vi "CRYCalc Constant Unit.vi"(6 "B_axis mode":u16(slide) scale=0.0..2.0, 7 "A_axis mode":u16(slide) scale=0.0..2.0, 8 "Work in":u16(slide), 9 "Operator":u16(ring) items=["+", "--", "x", "/"], 10 "B data for units":T1={"Name"="", "Curve"=[], "X data"=1, "Y data"=1, "Z data"=1, "X axis"=0, "Y axis"=1, "Z axis"=1, "X unit"="Hz", "Y unit"="", "Z unit"="deg.", "X dB ref"=1.0, "Y dB ref"=1.0, "Z dB ref"=1.0, "single val"=FALSE, "protected"=FALSE, "display X"=TRUE, "display Y"=TRUE, "display Z"=TRUE, "Test Info"="", "Step No."=0, "Plot Settings"={"Color"=0, "Interpolation"=0, "Point Style"=0, "Line Style"=0, "Point Color"=0, "Line Width"=0, "Bar Plot Style"=0, "Fill To"=0}, "AutoProtect"=FALSE} {"Z data" items=["dB", "Lin"]; "X data" items=["dB", "Lin"]; "Y data" items=["dB", "Lin"]; "Z dB ref" format="%.1f"; "Z axis" items=["Log", "Lin"]; "X dB ref" format="%.1f"; "X axis" items=["Log", "Lin"]; "Y axis" items=["Log", "Lin"]; "Y dB ref" format="%.1f"; "Curve"."z" format="%.2f"; "Curve"."y" format="%.2f"; "Curve"."x" format="%.2f"}, 11 "A data for units":T1={"Name"="", "Curve"=[], "X data"=1, "Y data"=1, "Z data"=1, "X axis"=0, "Y axis"=1, "Z axis"=1, "X unit"="Hz", "Y unit"="", "Z unit"="deg.", "X dB ref"=1.0, "Y dB ref"=1.0, "Z dB ref"=1.0, "single val"=FALSE, "protected"=FALSE, "display X"=TRUE, "display Y"=TRUE, "display Z"=TRUE, "Test Info"="", "Step No."=0, "Plot Settings"={"Color"=0, "Interpolation"=0, "Point Style"=0, "Line Style"=0, "Point Color"=0, "Line Width"=0, "Bar Plot Style"=0, "Fill To"=0}, "AutoProtect"=FALSE} {"Z data" items=["dB", "Lin"]; "X data" items=["dB", "Lin"]; "Y data" items=["dB", "Lin"]; "Z dB ref" format="%.1f"; "Z axis" items=["Log", "Lin"]; "X dB ref" format="%.1f"; "X axis" items=["Log", "Lin"]; "Y axis" items=["Log", "Lin"]; "Y dB ref" format="%.1f"; "Curve"."z" format="%.2f"; "Curve"."y" format="%.2f"; "Curve"."x" format="%.2f"}) -> (3 "Result out":T1={"Name"="", "Curve"=[], "X data"=1, "Y data"=1, "Z data"=1, "X axis"=0, "Y axis"=1, "Z axis"=1, "X unit"="Hz", "Y unit"="", "Z unit"="deg.", "X dB ref"=1.0, "Y dB ref"=1.0, "Z dB ref"=1.0, "single val"=FALSE, "protected"=FALSE, "display X"=TRUE, "display Y"=TRUE, "display Z"=TRUE, "Test Info"="", "Step No."=0, "Plot Settings"={"Color"=0, "Interpolation"=0, "Point Style"=0, "Line Style"=0, "Point Color"=0, "Line Width"=0, "Bar Plot Style"=0, "Fill To"=0}, "AutoProtect"=FALSE} {"Z data" items=["dB", "Lin"]; "X data" items=["dB", "Lin"]; "Y data" items=["dB", "Lin"]; "Z dB ref" format="%.1f"; "Z axis" items=["Log", "Lin"]; "X dB ref" format="%.1f"; "X axis" items=["Log", "Lin"]; "Y axis" items=["Log", "Lin"]; "Y dB ref" format="%.1f"; "Curve"."z" format="%.2f"; "Curve"."y" format="%.2f"; "Curve"."x" format="%.2f"})   [LabVIEW 2013]
uses:
  Typedef Control/CRYData Cluster.ctl
  CRYPost Processing Global.vi
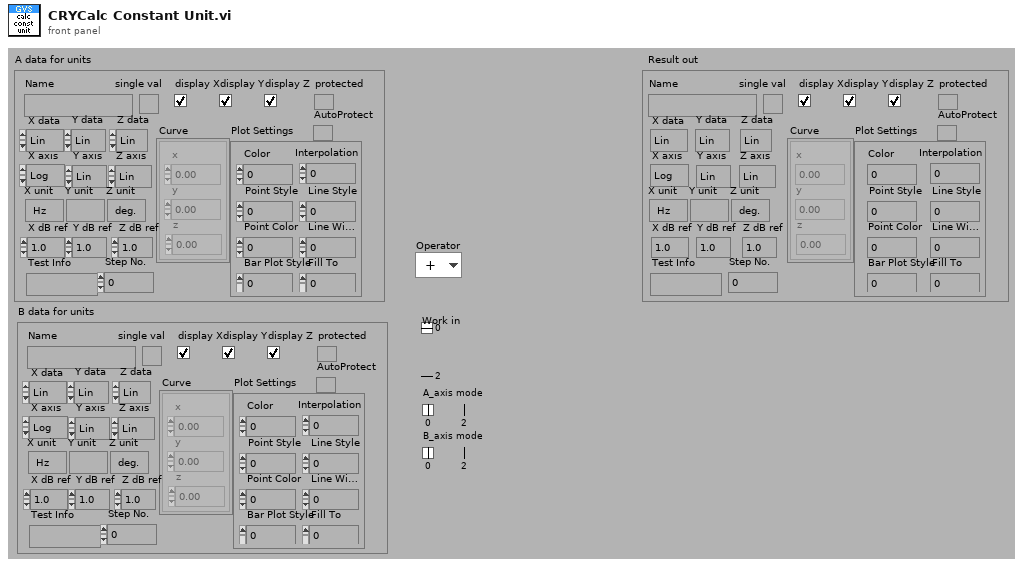
[diagram p1: front panel]
types:
  T1 = typedef "CRYData Cluster.ctl" = cluster{"Name":string, "Curve":cluster{"x":dbl, "y":dbl, "z":dbl}[], "X data":u16, "Y data":u16, "Z data":u16, "X axis":u16, "Y axis":u16, "Z axis":u16, "X unit":string, "Y unit":string, "Z unit":string, "X dB ref":dbl, "Y dB ref":dbl, "Z dB ref":dbl, "single val":bool, "protected":bool, "display X":bool, "display Y":bool, "display Z":bool, "Test Info":string, "Step No.":i32, "Plot Settings":cluster{"Color":u32, "Interpolation":u8, "Point Style":u8, "Line Style":u8, "Point Color":u32, "Line Width":u8, "Bar Plot Style":u8, "Fill To":i16}, "AutoProtect":bool}
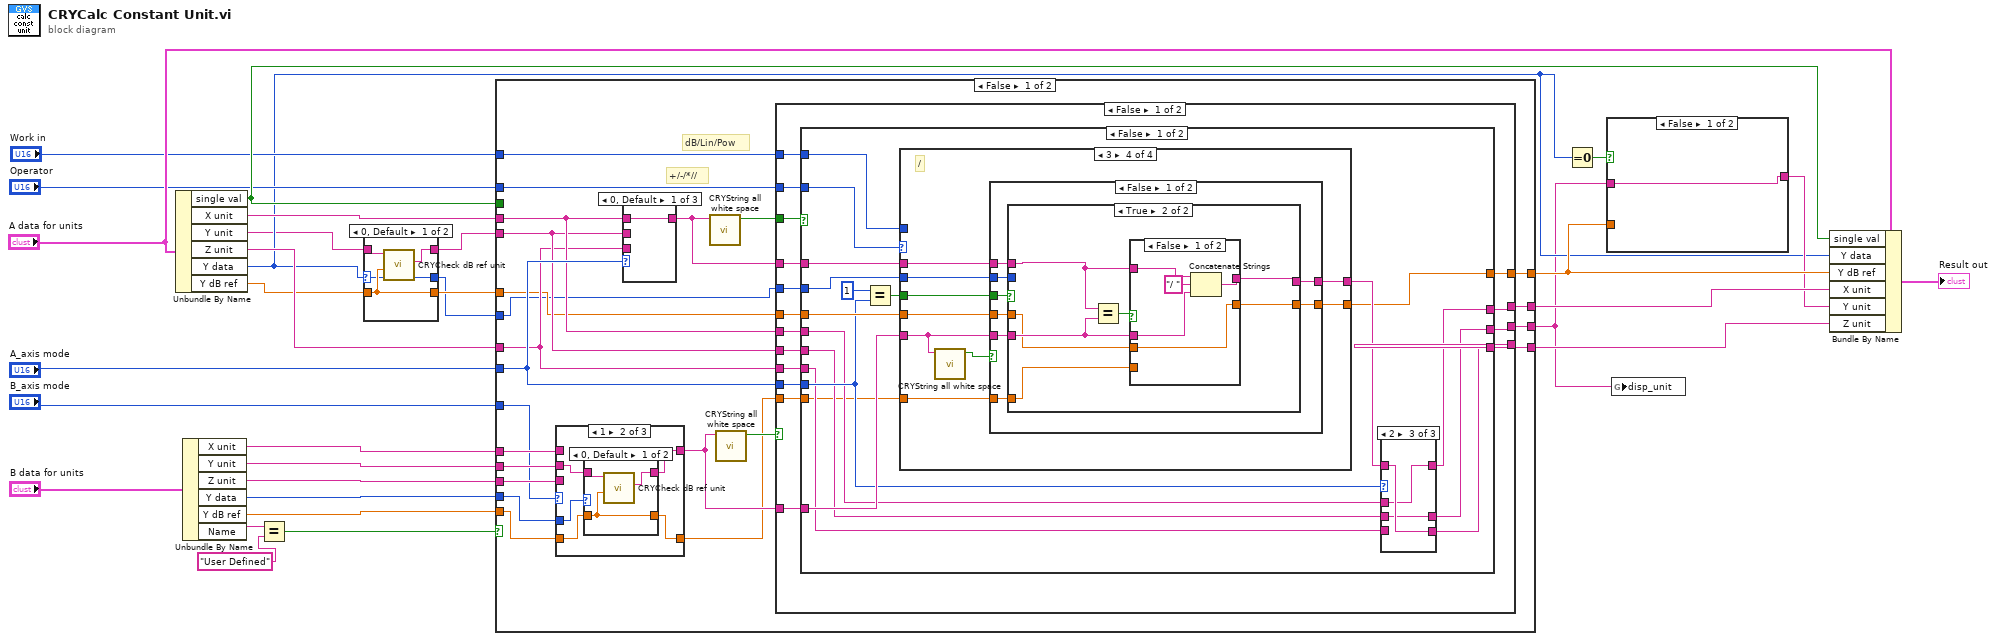
[diagram p0: block diagram]
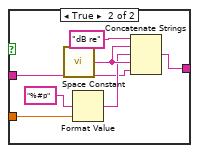
[diagram p3: hidden frame]
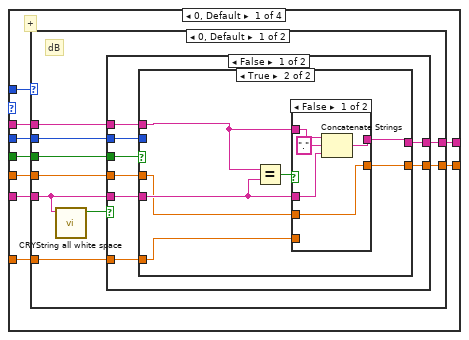
[diagram p9: hidden frame]
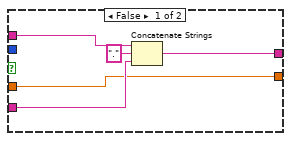
[diagram p10: hidden frame]
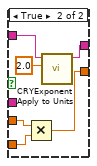
[diagram p11: hidden frame]
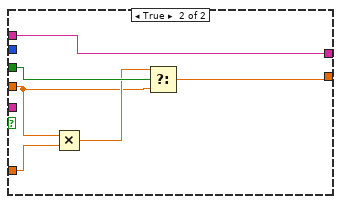
[diagram p12: hidden frame]
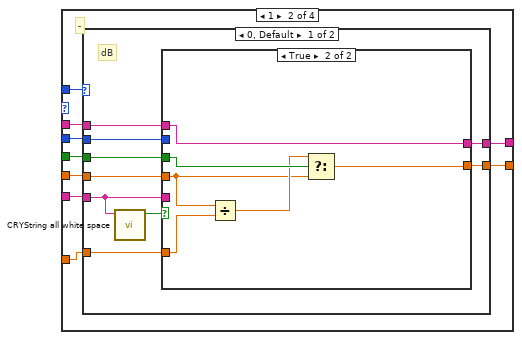
[diagram p14: hidden frame]
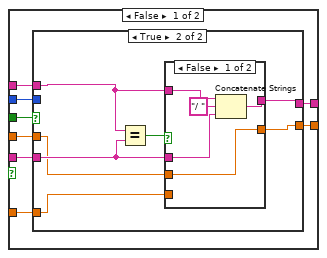
[diagram p15: hidden frame]
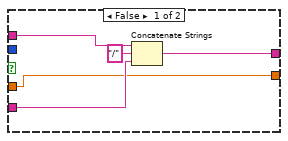
[diagram p16: hidden frame]
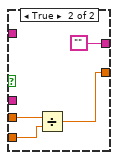
[diagram p17: hidden frame]
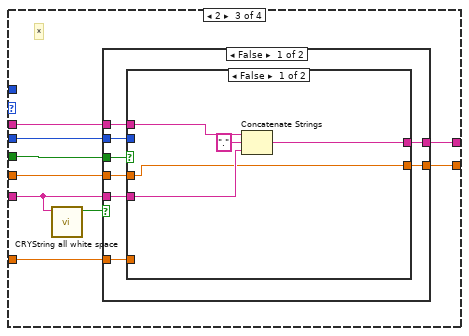
[diagram p19: hidden frame]
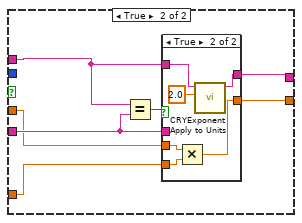
[diagram p20: hidden frame]
diagram:
  n1 = Unbundle By Name("A data for units") -> ("single val"=w22:bool, "X unit"=w29:string, "Y unit"=w3:string, "Z unit"=w8:string, "Y data"=w6:u16, "Y dB ref"=w7:dbl)
  n2 = Unbundle By Name("B data for units") -> ("X unit"=w28:string, "Y unit"=w30:string, "Z unit"=w27:string, "Y data"=w20:u16, "Y dB ref"=w19:dbl, "Name"=w25:string)
  n3 = Equal?(x=w25, y="User Defined") -> (x = y?=w21:bool)
  n4 = case shown="0, Default" w6 {
    selector: w6 -> [w31 w35]
    tunnel: w3 -> [w34 w37]
    tunnel: [w33 w37] -> w2
    tunnel: w7 -> [w32 w36]
    tunnel: [w32 w36] -> w5
    tunnel: [w31 w35] -> w4
    frame 0, Default {
      n5 = call "CRYCheck dB ref unit.vi"("dB ref in"=w32, "Unit in"=w34) -> ("Lin unit out"=w33:string)  [unwired: 9 out]
    }
    frame 1 {
    }
  }
  n6 = case shown="False" w21 {
    tunnel: w2 -> [w57 w345]
    tunnel: "Operator" -> [w49 _]
    tunnel: "Work in" -> [w50 _]
    tunnel: w22 -> [_ _]
    tunnel: w30 -> [w46 _]
    tunnel: "A_axis mode" -> [w59 _]
    tunnel: "B_axis mode" -> [w44 _]
    tunnel: w29 -> [w58 w348]
    tunnel: w8 -> [w56 w347]
    tunnel: w28 -> [w47 _]
    tunnel: w27 -> [w45 _]
    tunnel: [w53 w348] -> w24
    tunnel: [w55 w345] -> w1
    tunnel: [w54 w347] -> w23
    tunnel: w20 -> [w40 _]
    tunnel: w19 -> [w43 _]
    tunnel: w4 -> [w38 _]
    tunnel: [w48 w346] -> w10
    tunnel: w5 -> [w39 w346]
    frame False {
      # "+/-/*//"
      # "dB/Lin/Pow"
      n7 = case shown="1" w44 {
        tunnel: w47 -> [w62 _ _]
        tunnel: w46 -> [_ w66 _]
        tunnel: w45 -> [_ _ w74]
        tunnel: [w62 w64 w74] -> w42
        tunnel: w40 -> [_ w67 _]
        tunnel: w43 -> [w61 w65 w73]
        tunnel: [w61 w63 w73] -> w41
        frame 0, Default {
        }
        frame 1 {
          n8 = case shown="0, Default" w67 {
            tunnel: w66 -> [w70 w72]
            tunnel: [w69 w72] -> w64
            tunnel: w65 -> [w68 w71]
            tunnel: [w68 w71] -> w63
            frame 0, Default {
              n9 = call "CRYCheck dB ref unit.vi"("dB ref in"=w68, "Unit in"=w70) -> ("Lin unit out"=w69:string)  [unwired: 9 out]
            }
            frame 1 {
            }
          }
        }
        frame 2 {
        }
      }
      n10 = case shown="0, Default" w59 {
        tunnel: w58 -> [w342 _ _]
        tunnel: w57 -> [_ w343 _]
        tunnel: w56 -> [_ _ w344]
        tunnel: [w342 w343 w344] -> w51
        frame 0, Default {
        }
        frame 1 {
        }
        frame 2 {
        }
      }
      n11 = call "CRYString all white space.vi"("String"=w51) -> ("Nothing but white space?"=w52:bool)  [unwired: 10 in]
      n12 = call "CRYString all white space.vi"("String"=w42) -> ("Nothing but white space?"=w60:bool)  [unwired: 10 in]
      n13 = case shown="False" w60 {
        tunnel: w59 -> [w90 _]
        tunnel: w58 -> [w85 w341]
        tunnel: w57 -> [w89 w338]
        tunnel: w56 -> [w88 w340]
        tunnel: [w87 w338] -> w55
        tunnel: [w86 w340] -> w54
        tunnel: [w83 w341] -> w53
        tunnel: w42 -> [w84 _]
        tunnel: w52 -> [w82 _]
        tunnel: w51 -> [w81 _]
        tunnel: w50 -> [w80 _]
        tunnel: w49 -> [w79 _]
        tunnel: w38 -> [w78 _]
        tunnel: w39 -> [w77 w339]
        tunnel: [w76 w339] -> w48
        tunnel: w41 -> [w75 _]
        frame False {
          n14 = case shown="False" w82 {
            tunnel: w90 -> [w100 w328]
            tunnel: w89 -> [w98 w327]
            tunnel: w88 -> [w97 w326]
            tunnel: [w94 w325] -> w87
            tunnel: [w95 w324] -> w86
            tunnel: w85 -> [w99 w323]
            tunnel: w84 -> [w105 w322]
            tunnel: [w93 w321] -> w83
            tunnel: w81 -> [w106 _]
            tunnel: w80 -> [w107 _]
            tunnel: w79 -> [w108 _]
            tunnel: w78 -> [w102 _]
            tunnel: w77 -> [w101 w320]
            tunnel: [w92 w320] -> w76
            tunnel: w75 -> [w91 _]
            frame False {
              n15 = Equal?(x=u16 1, y=w100) -> (x = y?=w103:bool)
              n16 = case shown="3" w108 {
                tunnel: w107 -> [w126 w183 _ _]
                tunnel: w106 -> [w125 w182 w238 w284]
                tunnel: w105 -> [w124 w178 w231 w277]
                tunnel: w103 -> [w123 w180 w236 w282]
                tunnel: w102 -> [w122 w181 w237 w283]
                tunnel: [w121 w177 w234 w280] -> w96
                tunnel: w101 -> [w120 w179 w235 w281]
                tunnel: [w119 w176 w233 w279] -> w92
                tunnel: w91 -> [w118 w175 w232 w278]
                frame 0, Default {
                  # "+"
                  n17 = case shown="0, Default" w126 {
                    tunnel: w125 -> [w133 w174]
                    tunnel: w124 -> [w128 _]
                    tunnel: w123 -> [w135 _]
                    tunnel: w122 -> [w134 _]
                    tunnel: [w132 w174] -> w121
                    tunnel: w120 -> [w131 w173]
                    tunnel: [w130 w173] -> w119
                    tunnel: w118 -> [w129 _]
                    frame 0, Default {
                      # "dB"
                      n18 = call "CRYString all white space.vi"("String"=w128) -> ("Nothing but white space?"=w127:bool)  [unwired: 10 in]
                      n19 = case shown="False" w127 {
                        tunnel: w135 -> [w143 w170]
                        tunnel: w134 -> [w142 _]
                        tunnel: w133 -> [w141 w172]
                        tunnel: [w140 w172] -> w132
                        tunnel: w131 -> [w139 w168]
                        tunnel: [w138 w167] -> w130
                        tunnel: w129 -> [w137 w171]
                        tunnel: w128 -> [w136 _]
                        frame False {
                          n20 = case shown="True" w143 {
                            tunnel: w142 -> [_ _]
                            tunnel: w141 -> [w148 w155]
                            tunnel: w136 -> [w147 w154]
                            tunnel: [w145 w153] -> w140
                            tunnel: w139 -> [w144 w152]
                            tunnel: [w144 w151] -> w138
                            tunnel: w137 -> [_ w150]
                            frame False {
                              n21 = Concatenate Strings(w148, "." ("string"), w147) -> (w145:string)
                            }
                            frame True {
                              n22 = Equal?(x=w155, y=w154) -> (x = y?=w149:bool)
                              n23 = case shown="False" w149 {
                                tunnel: w155 -> [w159 w165]
                                tunnel: [w160 w164] -> w153
                                tunnel: w154 -> [w157 _]
                                tunnel: w152 -> [w156 w163]
                                tunnel: [w156 w161] -> w151
                                tunnel: w150 -> [_ w162]
                                frame False {
                                n24 = Concatenate Strings(w159, "." ("string"), w157) -> (w160:string)
                                }
                                frame True {
                                n25 = Multiply(x=w163, y=w162) -> (x*y=w161:dbl)
                                n26 = call "CRYExponent Apply to Units.vi"("Exponent to apply"=2.0, "Unit in"=w165) -> ("Unit out"=w164:string)  [unwired: 9 out]
                                }
                              }
                            }
                          }
                        }
                        frame True {
                          n27 = Multiply(x=w168, y=w171) -> (x*y=w169:dbl)
                          n28 = Select(t=w169, s=w170, f=w168) -> (s? t:f=w167:dbl)
                        }
                      }
                    }
                    frame 1, 2 {
                      # "Lin,Pow"
                    }
                  }
                }
                frame 1 {
                  # "-"
                  n29 = case shown="0, Default" w183 {
                    tunnel: w182 -> [w190 w229]
                    tunnel: w178 -> [w185 _]
                    tunnel: w180 -> [w192 _]
                    tunnel: w181 -> [w191 _]
                    tunnel: [w189 w229] -> w177
                    tunnel: w179 -> [w188 w228]
                    tunnel: [w187 w228] -> w176
                    tunnel: w175 -> [w186 _]
                    frame 0, Default {
                      # "dB"
                      n30 = call "CRYString all white space.vi"("String"=w185) -> ("Nothing but white space?"=w184:bool)  [unwired: 10 in]
                      n31 = case shown="True" w184 {
                        tunnel: w192 -> [w200 w225]
                        tunnel: w191 -> [w199 _]
                        tunnel: w190 -> [w198 w227]
                        tunnel: [w197 w227] -> w189
                        tunnel: w188 -> [w196 w223]
                        tunnel: [w195 w222] -> w187
                        tunnel: w186 -> [w194 w226]
                        tunnel: w185 -> [w193 _]
                        frame False {
                          n32 = case shown="True" w200 {
                            tunnel: w199 -> [_ _]
                            tunnel: w198 -> [w205 w212]
                            tunnel: w193 -> [w204 w211]
                            tunnel: [w202 w210] -> w197
                            tunnel: w196 -> [w201 w209]
                            tunnel: [w201 w208] -> w195
                            tunnel: w194 -> [_ w207]
                            frame False {
                              n33 = Concatenate Strings(w205, "/" ("string"), w204) -> (w202:string)
                            }
                            frame True {
                              n34 = Equal?(x=w212, y=w211) -> (x = y?=w206:bool)
                              n35 = case shown="False" w206 {
                                tunnel: w212 -> [w216 _]
                                tunnel: [w217 ""] -> w210
                                tunnel: w211 -> [w214 _]
                                tunnel: [w213 w218] -> w208
                                tunnel: w209 -> [w213 w220]
                                tunnel: w207 -> [_ w219]
                                frame False {
                                n36 = Concatenate Strings(w216, "/ " ("string"), w214) -> (w217:string)
                                }
                                frame True {
                                n37 = Divide(x=w220, y=w219) -> (x/y=w218:dbl)
                                }
                              }
                            }
                          }
                        }
                        frame True {
                          n38 = Divide(x=w223, y=w226) -> (x/y=w224:dbl)
                          n39 = Select(t=w224, s=w225, f=w223) -> (s? t:f=w222:dbl)
                        }
                      }
                    }
                    frame 1, 2 {
                      # "Lin,Pow"
                    }
                  }
                }
                frame 2 {
                  # "*"
                  n40 = call "CRYString all white space.vi"("String"=w231) -> ("Nothing but white space?"=w230:bool)  [unwired: 10 in]
                  n41 = case shown="False" w230 {
                    tunnel: w238 -> [w246 w275]
                    tunnel: w237 -> [w245 _]
                    tunnel: w236 -> [w244 w273]
                    tunnel: w235 -> [w243 w272]
                    tunnel: [w242 w275] -> w234
                    tunnel: [w241 w270] -> w233
                    tunnel: w232 -> [w240 w271]
                    tunnel: w231 -> [w239 _]
                    frame False {
                      n42 = case shown="False" w244 {
                        tunnel: w245 -> [_ _]
                        tunnel: w246 -> [w251 w258]
                        tunnel: w239 -> [w250 w257]
                        tunnel: [w248 w256] -> w242
                        tunnel: w243 -> [w247 w255]
                        tunnel: [w247 w254] -> w241
                        tunnel: w240 -> [_ w253]
                        frame False {
                          n43 = Concatenate Strings(w251, "." ("string"), w250) -> (w248:string)
                        }
                        frame True {
                          n44 = Equal?(x=w258, y=w257) -> (x = y?=w252:bool)
                          n45 = case shown="True" w252 {
                            tunnel: w258 -> [w262 w268]
                            tunnel: [w263 w267] -> w256
                            tunnel: w257 -> [w260 _]
                            tunnel: w255 -> [w259 w266]
                            tunnel: [w259 w264] -> w254
                            tunnel: w253 -> [_ w265]
                            frame False {
                              n46 = Concatenate Strings(w262, "." ("string"), w260) -> (w263:string)
                            }
                            frame True {
                              n47 = Multiply(x=w266, y=w265) -> (x*y=w264:dbl)
                              n48 = call "CRYExponent Apply to Units.vi"("Exponent to apply"=2.0, "Unit in"=w268) -> ("Unit out"=w267:string)  [unwired: 9 out]
                            }
                          }
                        }
                      }
                    }
                    frame True {
                      n49 = Multiply(x=w272, y=w271) -> (x*y=w274:dbl)
                      n50 = Select(t=w274, s=w273, f=w272) -> (s? t:f=w270:dbl)
                    }
                  }
                }
                frame 3 {
                  # "/"
                  n51 = call "CRYString all white space.vi"("String"=w277) -> ("Nothing but white space?"=w276:bool)  [unwired: 10 in]
                  n52 = case shown="False" w276 {
                    tunnel: w284 -> [w292 w319]
                    tunnel: w283 -> [w291 _]
                    tunnel: w282 -> [w290 w318]
                    tunnel: w281 -> [w289 w317]
                    tunnel: [w288 w319] -> w280
                    tunnel: [w287 w314] -> w279
                    tunnel: w278 -> [w286 w316]
                    tunnel: w277 -> [w285 _]
                    frame False {
                      n53 = case shown="True" w290 {
                        tunnel: w291 -> [_ _]
                        tunnel: w292 -> [w297 w304]
                        tunnel: w285 -> [w296 w303]
                        tunnel: [w294 w302] -> w288
                        tunnel: w289 -> [w293 w301]
                        tunnel: [w293 w299] -> w287
                        tunnel: w286 -> [_ w300]
                        frame False {
                          n54 = Concatenate Strings(w297, "/ " ("string"), w296) -> (w294:string)
                        }
                        frame True {
                          n55 = Equal?(x=w304, y=w303) -> (x = y?=w298:bool)
                          n56 = case shown="False" w298 {
                            tunnel: w304 -> [w308 _]
                            tunnel: [w309 ""] -> w302
                            tunnel: w303 -> [w306 _]
                            tunnel: w301 -> [w305 w312]
                            tunnel: w300 -> [_ w311]
                            tunnel: [w305 w310] -> w299
                            frame False {
                              n57 = Concatenate Strings(w308, "/ " ("string"), w306) -> (w309:string)
                            }
                            frame True {
                              n58 = Divide(x=w312, y=w311) -> (x/y=w310:dbl)
                            }
                          }
                        }
                      }
                    }
                    frame True {
                      n59 = Divide(x=w317, y=w316) -> (x/y=w315:dbl)
                      n60 = Select(t=w315, s=w318, f=w317) -> (s? t:f=w314:dbl)
                    }
                  }
                }
              }
              n61 = case shown="2" w100 {
                tunnel: w99 -> [_ w113 w115]
                tunnel: w98 -> [w111 _ w116]
                tunnel: w97 -> [w110 w112 _]
                tunnel: w96 -> [w109 w114 w117]
                tunnel: [w111 w114 w116] -> w94
                tunnel: [w110 w112 w117] -> w95
                tunnel: [w109 w113 w115] -> w93
                frame 0, Default {
                }
                frame 1 {
                }
                frame 2 {
                }
              }
            }
            frame True {
              n62 = case shown="2" w328 {
                tunnel: w323 -> [_ w334 w336]
                tunnel: w327 -> [w331 _ w337]
                tunnel: w326 -> [w330 w333 _]
                tunnel: [w331 w332 w337] -> w325
                tunnel: [w330 w333 w335] -> w324
                tunnel: [w329 w334 w336] -> w321
                tunnel: w322 -> [w329 w332 w335]
                frame 0, Default {
                }
                frame 1 {
                }
                frame 2 {
                }
              }
            }
          }
        }
        frame True {
        }
      }
    }
    frame True {
      # "Constant"
    }
  }
  n63 = Equal To 0?(x=w6) -> (x = 0?=w11:bool)
  n64 = case shown="False" w11 {
    tunnel: w1 -> [w349 w351]
    tunnel: [w349 w350] -> w9
    tunnel: w10 -> [_ w355]
    frame False {
    }
    frame True {
      n65 = call <vilib>:"Space Constant.vi"() -> ("String"=w354:string)
      n66 = Format Value(format string="%#p", value (0)=w355) -> (output string=w352:string)  [unwired: 1 out]
      n67 = Concatenate Strings("dB re" ("string"), w354, w352, w354, w351) -> (w350:string)
    }
  }
  n68 = global write "CRYPost Processing Global.vi" "disp_unit"(w1) -> ()
  n69 = Bundle By Name(cluster="A data for units", "single val"=w22, "Y data"=w6, "Y dB ref"=w10, "X unit"=w24, "Y unit"=w9, "Z unit"=w23) -> (→"Result out":T1)
